vi "DFD Build Filter from Transfer Function.vi"(6 "fs [Hz]":dbl=1.0 format="%#_2g", 8 "error in (no error)":errorcluster, 9 "denominator":dbl[](array[numeric])=[1.0], 10 "numerator":dbl[](array[numeric])) -> (0 "error out":errorcluster, 3 "filter out":T1={"mSRate_Fs"=1.0, "mSRate_Version"="2.0", "mSRate_Comments"="", "mSRate_OrgCoef"={"type"=enum."Undefined", "gain"=1.0, "coef a (k)"=[], "coef b (v)"=[]}, "mSRate_CurCoef"={"type"=enum."Undefined", "gain"=1.0, "coef a (k)"=[], "coef b (v)"=[]}, "mSRate_Quantized?"=FALSE, "mSRate_QCoef"={"type"=enum."Undefined", "gain"=1.0, "coef a (k)"=[], "coef b (v)"=[]}, "mSRate_QSettings"=[], "mSRate_Order"=0, "mSRate_Scaling"={"mSRate_ScaleByPowerOf2?"=FALSE, "mSRate_ScaleType"=enum."No Norm"}} {"mSRate_QSettings"."source" items=["Coef a/k"=0, "Coef b/v"=7, "Input"=1, "Output"=2, "Multiplicand"=3, "Product"=4, "Sum"=5, "Delay"=6, "Gain"=8]})   [LabVIEW 2017, in "NI_DigFilterLicensed.lvlib"]
doc: "Creates a filter from a transfer function."
uses:
  <vilib>/addons/Digital Filter Design/NI_DigFilterLicensed.lvlib
  <vilib>/addons/Digital Filter Design/_Objects.llb/DFD Filter Obj.ctl
  <vilib>/addons/Digital Filter Design/_Objects.llb/DFD Filter Coef.ctl
  <vilib>/addons/Digital Filter Design/_Objects.llb/DFD Filter Structure Type Selector.ctl
  <vilib>/addons/Digital Filter Design/_Objects.llb/dfd_Internal Quantization Settings.ctl
  <vilib>/addons/Digital Filter Design/_Objects.llb/dfd_Internal Quantization Srcs.ctl
  <vilib>/addons/Digital Filter Design/_Objects.llb/DFD Coef Norm Type.ctl
panel:
  in  "filter in":T1={"mSRate_Fs"=1.0, "mSRate_Version"="2.0", "mSRate_Comments"="", "mSRate_OrgCoef"={"type"=enum."Undefined", "gain"=1.0, "coef a (k)"=[], "coef b (v)"=[]}, "mSRate_CurCoef"={"type"=enum."Undefined", "gain"=1.0, "coef a (k)"=[], "coef b (v)"=[]}, "mSRate_Quantized?"=FALSE, "mSRate_QCoef"={"type"=enum."Undefined", "gain"=1.0, "coef a (k)"=[], "coef b (v)"=[]}, "mSRate_QSettings"=[], "mSRate_Order"=0, "mSRate_Scaling"={"mSRate_ScaleByPowerOf2?"=FALSE, "mSRate_ScaleType"=enum."No Norm"}} {"mSRate_QSettings"."source" items=["Coef a/k"=0, "Coef b/v"=7, "Input"=1, "Output"=2, "Multiplicand"=3, "Product"=4, "Sum"=5, "Delay"=6, "Gain"=8]}
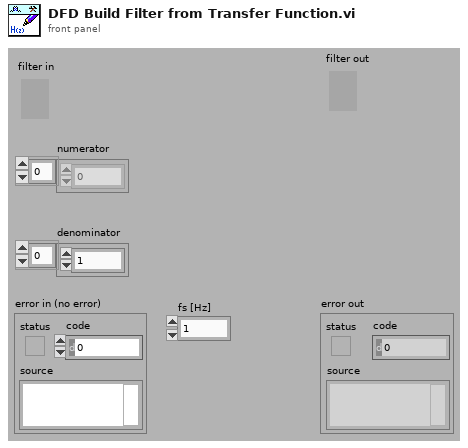
[diagram p1: front panel]
types:
  T1 = typedef "NI_DigFilterLicensed.lvlib/DFD Filter Obj.ctl" = cluster{"mSRate_Fs":dbl, "mSRate_Version":string, "mSRate_Comments":string, "mSRate_OrgCoef":T2, "mSRate_CurCoef":T2, "mSRate_Quantized?":bool, "mSRate_QCoef":T2, "mSRate_QSettings":T4[], "mSRate_Order":i32, "mSRate_Scaling":cluster{"mSRate_ScaleByPowerOf2?":bool, "mSRate_ScaleType":T6}}
  T2 = typedef "NI_DigFilterLicensed.lvlib/DFD Filter Coef.ctl" = cluster{"type":T3, "gain":dbl, "coef a (k)":dbl[], "coef b (v)":dbl[]}
  T3 = typedef "NI_DigFilterLicensed.lvlib/DFD Filter Structure Type Selector.ctl" = enum16{"Undefined", "FIR Direct Form", "FIR Direct Form Transposed", "FIR Symmetric", "FIR Antisymmetric", "IIR Direct Form I", "IIR Direct Form I Transposed", "IIR Direct Form II", "IIR Direct Form II Transposed", "IIR Cascaded Second Order Sections Form I", "IIR Cascaded Second Order Sections Form I Transposed", "IIR Cascaded Second Order Sections Form II", "IIR Cascaded Second Order Sections Form II Transposed", "Lattice Allpass (basic sections)", "Lattice Allpass (one multiplier sections)", "Lattice Allpass (normalized sections)", "Lattice AR (basic sections)", "Lattice AR (one multiplier sections)", "Lattice AR (normalized sections)", "Lattice MA (minimum phase)", "Lattice MA (maximum phase)", "Lattice ARMA (basic sections)", "Lattice ARMA (one multiplier sections)", "Lattice ARMA (normalized sections)"}
  T4 = typedef "NI_DigFilterLicensed.lvlib/dfd_Internal Quantization Settings.ctl" = cluster{"source":T5, "wl":i16, "iwl":i16, "overflow mode":enum16{"Saturation", "Wrap"}, "rounding mode":enum16{"Nearest", "Truncation"}, "signed?":bool}
  T5 = typedef "NI_DigFilterLicensed.lvlib/dfd_Internal Quantization Srcs.ctl" = u16
  T6 = typedef "NI_DigFilterLicensed.lvlib/DFD Coef Norm Type.ctl" = enum16{"No Norm", "Time Domain 1-Norm", "Time Domain 2-Norm", "Time Domain Inf-Norm"}
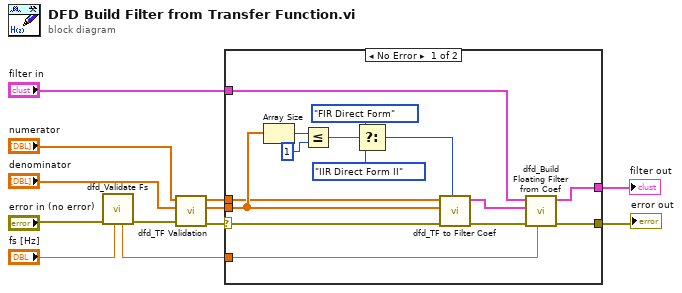
[diagram p0: block diagram]
diagram:
  n1 = call <vilib>:"dfd_Validate Fs.vi"("fs [Hz]"="fs [Hz]", "error in (no error)"="error in (no error)") -> ("error out"=w3:errorcluster, "dup fs [Hz]"=w2:dbl)  [unwired: 8 in]
  n2 = call <vilib>:"dfd_TF Validation.vi"("error in (no error)"=w3, "denominator"="denominator", "numerator"="numerator") -> ("error out"=w9:errorcluster, "validated denominator"=w7:dbl[], "validated numerator"=w8:dbl[])  [unwired: 3 out]
  n3 = case shown="No Error" w9 {
    selector: w9 -> [w21 w29]
    tunnel: [w14 w29] -> w12
    tunnel: "filter in" -> [w18 w28]
    tunnel: w8 -> [w17 _]
    tunnel: w7 -> [w22 _]
    tunnel: [w15 w28] -> w5
    tunnel: w2 -> [w13 _]
    frame No Error {
      n4 = Array Size(array=w22) -> (size(s)=w16:i32)
      n5 = Less Or Equal?(x=w16, y=1) -> (x <= y?=w26:bool)
      n6 = Select(t=DFD_Filter_Structure_Type_Selector."FIR Direct Form" ("struct typ"), s=w26, f=DFD_Filter_Structure_Type_Selector."IIR Direct Form II" ("struct typ")) -> (s? t:f=w23:T3)
      n7 = call <vilib>:"dfd_TF to Filter Coef.vi"("type"=w23, "error in (no error)"=w21, "denominator"=w22, "numerator"=w17) -> ("error out"=w20:errorcluster, "filter coef"=w19:T2)  [unwired: 6 out]
      n8 = call <vilib>:"dfd_Build Floating Filter from Coef.vi"("fs [Hz]"=w13, "error in (no error)"=w20, "filter coef"=w19, "filter in"=w18) -> ("error out"=w14:errorcluster, "filter out"=w15:T1)  [unwired: 6 out]
    }
    frame Error {
    }
  }
  "filter out" <- w5
  "error out" <- w12
